vi "Graphics-Autoscale Y.vi"(0 "XYGraph in":refnum<vi>, 1 "Value":cluster{"Freq (kHz)":dbl[], "Avg Mag":dbl[]}[](array[cluster]), 5 "Autoscale mode":enum16{"Off", "Min", "Max", "All"}(ring)=enum."All", 7 "Xmin":dbl=nan, 9 "Xmax":dbl=nan, 11 "error in (no error)":errorcluster, 12 "Resolution":dbl) -> (4 "XYGraph out":refnum<vi>, 15 "error out":errorcluster)   [LabVIEW 2020]
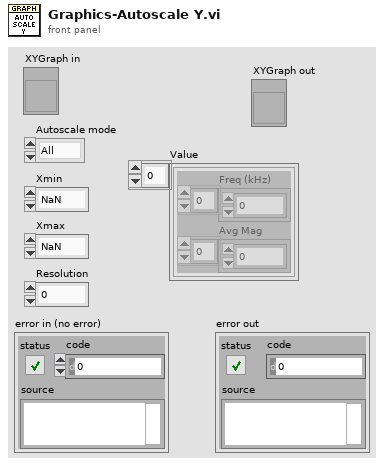
[diagram p1: front panel]
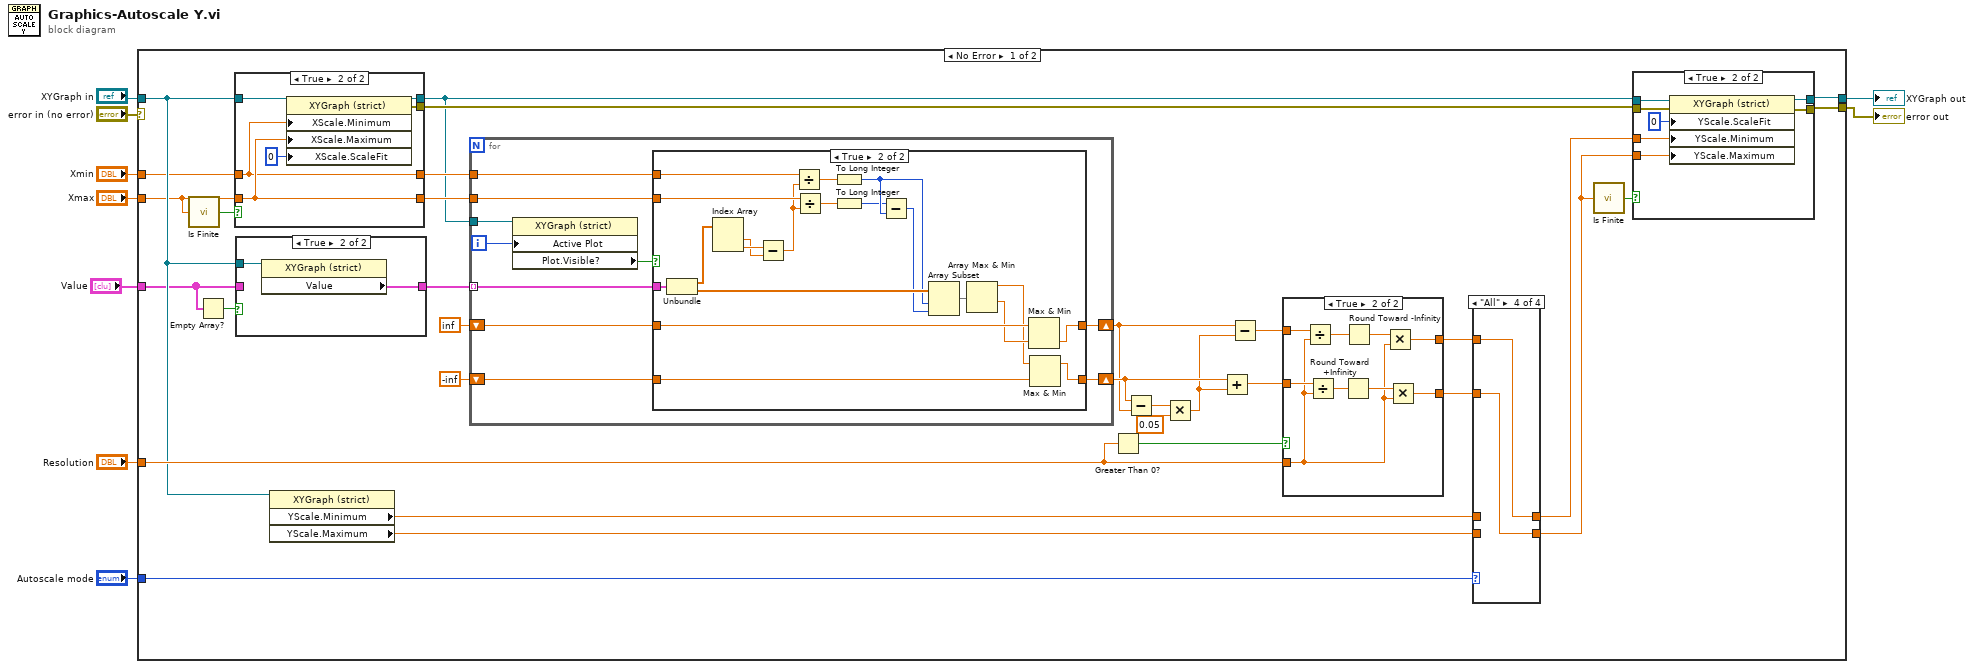
[diagram p0: block diagram]
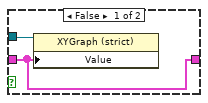
[diagram p2: hidden frame]
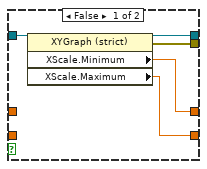
[diagram p3: hidden frame]
diagram:
  n1 = case shown="No Error" "error in (no error)" {
    selector: "error in (no error)" -> [_ w118]
    tunnel: "XYGraph in" -> [w28 w117]
    tunnel: [w37 w118] -> w8
    tunnel: [w38 w117] -> w6
    tunnel: "Resolution" -> [w36 _]
    tunnel: "Autoscale mode" -> [w34 _]
    tunnel: "Xmin" -> [w26 _]
    tunnel: "Xmax" -> [w21 _]
    tunnel: "Value" -> [w24 _]
    frame No Error {
      n2 = call "Is Finite.vi"("Numeric"=w21) -> ("is finite?"=w20:bool)
      n3 = Empty Array?(array=w24) -> (empty?=w25:bool)
      n4 = case shown="True" w20 {
        tunnel: [w50 w52] -> w41
        tunnel: [w49 w53] -> w40
        tunnel: [w48 w55] -> w17
        tunnel: [w47 w54] -> w39
        tunnel: w28 -> [w46 w56]
        tunnel: w26 -> [_ w52]
        tunnel: w21 -> [_ w53]
        frame False {
          n5 = property class="XYGraph (strict)"(reference=w46) -> (reference out=w48:refnum<vi>, error out=w47:errorcluster, "XScale.Minimum"=w50:dbl, "XScale.Maximum"=w49:dbl)  [unwired: 1 in]
        }
        frame True {
          n6 = property class="XYGraph (strict)"(reference=w56, "XScale.Minimum"=w52, "XScale.Maximum"=w53, "XScale.ScaleFit"=u8 0 ("X Scale.Scale Fit")) -> (reference out=w55:refnum<vi>, error out=w54:errorcluster)  [unwired: 1 in]
        }
      }
      n7 = case shown="True" w25 {
        tunnel: w28 -> [w43 w45]
        tunnel: [w42 w44] -> w27
        tunnel: w24 -> [w42 _]
        frame False {
          n8 = property class="XYGraph (strict)"(reference=w43, "Value"=w42) -> ()  [unwired: 1 in, 2 out]
        }
        frame True {
          n9 = property class="XYGraph (strict)"(reference=w45) -> ("Value"=w44:cluster{"Freq (kHz)":dbl[], "Avg Mag":dbl[]}[])  [unwired: 1 in, 2 out]
        }
      }
      n10 = property class="XYGraph (strict)"(reference=w28) -> ("YScale.Minimum"=w33:dbl, "YScale.Maximum"=w32:dbl)  [unwired: 1 in, 2 out]
      n11 = for {
        tunnel: w27 -> [w66] mode=indexing
        tunnel: w41 -> [w61]
        tunnel: w40 -> [w60]
        shift-right: [w63] -> w15
        shift-left: inf -> [w64]
        shift-right: [w62] -> w16
        shift-left: -inf -> [w65]
        tunnel: w17 -> [w57]
        i -> [w58]
        n12 = property class="XYGraph (strict)"(reference=w57, "Active Plot"=w58) -> ("Plot.Visible?"=w59:bool)  [unwired: 1 in, 2 out]
        n13 = case shown="True" w59 {
          tunnel: w66 -> [_ w88]
          tunnel: w65 -> [w67 w84]
          tunnel: w64 -> [w68 w83]
          tunnel: [w68 w82] -> w63
          tunnel: [w67 w81] -> w62
          tunnel: w61 -> [_ w77]
          tunnel: w60 -> [_ w76]
          frame False {
          }
          frame True {
            n14 = Unbundle(w88) -> ("Freq (kHz)"=w80:dbl[], "Avg Mag"=w87:dbl[])
            n15 = Index Array(array=w80) -> (element #1=w78:dbl, element #2=w79:dbl)  [unwired: 2 in]
            n16 = Subtract(x=w79, y=w78) -> (x-y=w75:dbl)
            n17 = Divide(x=w77, y=w75) -> (x/y=w74:dbl)
            n18 = Divide(x=w76, y=w75) -> (x/y=w73:dbl)
            n19 = To Long Integer(number=w74) -> (32bit integer=w72:i32)
            n20 = To Long Integer(number=w73) -> (32bit integer=w71:i32)
            n21 = Subtract(x=w71, y=w72) -> (x-y=w86:i32)
            n22 = Array Subset(array=w87, index=w72, length=w86) -> (w85:dbl[])
            n23 = Array Max & Min(array=w85) -> (max value=w69:dbl, min value=w70:dbl)  [unwired: 2 out]
            n24 = Max & Min(x=w83, y=w70) -> (min(x,y)=w82:dbl)  [unwired: 1 out]
            n25 = Max & Min(x=w69, y=w84) -> (max(x,y)=w81:dbl)  [unwired: 1 out]
          }
        }
      }
      n26 = Greater Than 0?(x=w36) -> (x > 0?=w35:bool)
      n27 = Subtract(x=w16, y=w15) -> (x-y=w14:dbl)
      n28 = Multiply(x=w14, y=0.05) -> (x*y=w10:dbl)
      n29 = Add(x=w16, y=w10) -> (x+y=w12:dbl)
      n30 = Subtract(x=w15, y=w10) -> (x-y=w11:dbl)
      n31 = case shown="True" w35 {
        tunnel: w11 -> [w98 w107]
        tunnel: w12 -> [w97 w104]
        tunnel: [w98 w101] -> w30
        tunnel: [w97 w100] -> w29
        tunnel: w36 -> [_ w99]
        frame False {
        }
        frame True {
          n32 = Divide(x=w107, y=w99) -> (x/y=w106:dbl)
          n33 = Divide(x=w104, y=w99) -> (x/y=w103:dbl)
          n34 = Round Toward +Infinity(x=w103) -> (ceil(x): smallest int >= x=w102:dbl)
          n35 = Round Toward -Infinity(1:w106) -> (0:w105:dbl)
          n36 = Multiply(x=w105, y=w99) -> (x*y=w101:dbl)
          n37 = Multiply(x=w102, y=w99) -> (x*y=w100:dbl)
        }
      }
      n38 = case shown="\"All\"" w34 {
        tunnel: w33 -> [w90 _ w94 _]
        tunnel: w32 -> [w89 w92 _ _]
        tunnel: [w90 w91 w94 w96] -> w31
        tunnel: [w89 w92 w93 w95] -> w23
        tunnel: w30 -> [_ w91 _ w96]
        tunnel: w29 -> [_ _ w93 w95]
        frame "Off", Default {
        }
        frame "Min" {
        }
        frame "Max" {
        }
        frame "All" {
        }
      }
      n39 = call "Is Finite.vi"("Numeric"=w23) -> ("is finite?"=w22:bool)
      n40 = case shown="True" w22 {
        tunnel: w17 -> [w109 w116]
        tunnel: w39 -> [w108 w115]
        tunnel: [w109 w114] -> w38
        tunnel: [w108 w113] -> w37
        tunnel: w31 -> [_ w111]
        tunnel: w23 -> [_ w110]
        frame False {
        }
        frame True {
          n41 = property class="XYGraph (strict)"(reference=w116, error in=w115, "YScale.ScaleFit"=u8 0 ("Y Scale.Scale Fit"), "YScale.Minimum"=w111, "YScale.Maximum"=w110) -> (reference out=w114:refnum<vi>, error out=w113:errorcluster)
        }
      }
    }
    frame Error {
    }
  }
  "error out" <- w8
  "XYGraph out" <- w6
